vi "SPD.Config Read Test07 TR bifurcation.vi"(8 "Error In":errorcluster, 11 "SPD.Stand Ctrl in":T2 {"spdDeviceSession"."hidSPD.Sturtup Values"."HV_bias" format="%#_6p, V"; "spdDeviceSession"."hidSPD.Sturtup Values"."TSet" format="%#_6p, DegC"; "spdDeviceSession"."hidSPD.Controller"."HV_bias" format="%#_6p, V"; "spdDeviceSession"."hidSPD.Controller"."TSet" format="%#_6p, DegC"}) -> (0 "Error Out":errorcluster, 2 "TR_Bif Meas Params":T1, 3 "SPD.Stand Ctrl out":T2 {"spdDeviceSession"."hidSPD.Sturtup Values"."HV_bias" format="%#_6p, V"; "spdDeviceSession"."hidSPD.Sturtup Values"."TSet" format="%#_6p, DegC"; "spdDeviceSession"."hidSPD.Controller"."HV_bias" format="%#_6p, V"; "spdDeviceSession"."hidSPD.Controller"."TSet" format="%#_6p, DegC"})   [LabVIEW 2018]
uses:
  typedefs/SPD.Stand Ctrl.ctl
  Instruments/SPD HID Interface/hidSPDLibForLabView/LibVIs/hidSPD Controls/hidSPD Device Session.ctl
  Instruments/SPD HID Interface/hidSPDLibForLabView/LibVIs/hidSPD Controls/hidSPD Controller.ctl
  Instruments/SPD HID Interface/hidSPDLibForLabView/LibVIs/hidSPD Controls/hidSPD SPD Type.ctl
  Instruments/KC705 DevBoard/typedefs/DevB.Session.ctl
  Instruments/KeySight 53230A/typedefs/FreqC.Session.ctl
  Instruments/KeySight 8164B/KeySight 8164B LAN InstrLib/typedefs/KeySight 8164B control.ctl
  Instruments/LeCroy SDA830/typedefs/LeCroy.Session.ctl
  typedefs/SPD.Events.ctl
  SPD.Config File ctrl.ctl
  <vilib>/Utility/config.llb/Config Data RefNum.ctl
  typedefs/SPD.Meas Result.ctl
  typedefs/SPD.Queues.ctl
  typedefs/SPD.Stand state.ctl
  SPD Measurements/TR Bifurcation/typedefs/SPD.TR Test Params.ctl
  <vilib>/Utility/config.llb/Read Key (I32).vi
  <vilib>/Utility/config.llb/Read Key (Double).vi
  <vilib>/Utility/config.llb/Read Key (String).vi
  <vilib>/Utility/config.llb/NI_LVConfig.lvlib
  Instruments/KeySight 8164B/KeySight 8164B LAN InstrLib.lvlib
  Instruments/SPD HID Interface/hidSPDLibForLabView/hidSPDLibForLabView.lvlib
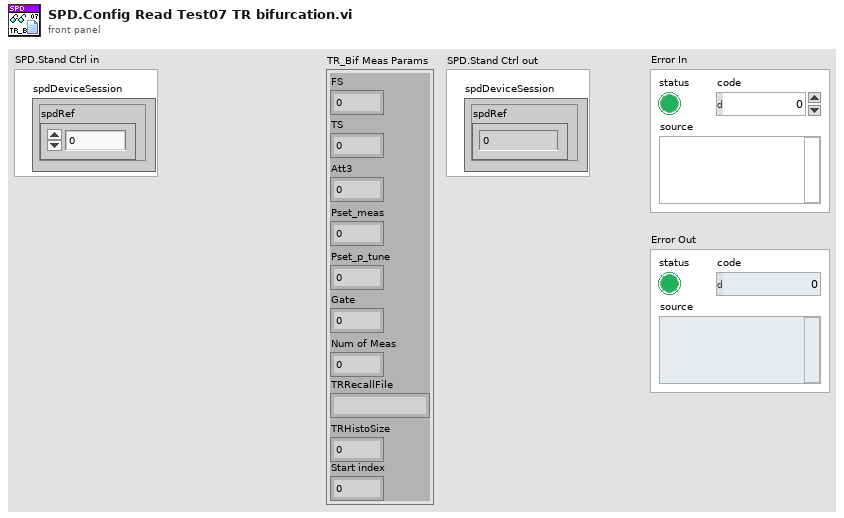
[diagram p1: front panel]
types:
  T1 = typedef "SPD.TR Test Params.ctl" = cluster{"FS":i32, "TS":i32, "Att3":dbl, "Pset_meas":dbl, "Pset_p_tune":dbl, "Gate":dbl, "Num of Meas":i32, "TRRecallFile":string, "TRHistoSize":i32, "Start index":i32}
  T2 = typedef "SPD.Stand Ctrl.ctl" = cluster{"spdDeviceSession":T3, "DevBSession":T6, "FreqCSession":T7, "8164BSession":T8, "LeCroySession":T9, "Events":T10, "configFile":T11, "SPD.Result":T13, "SPD.Queues":T14, "Console":refnum<vi>}
  T3 = typedef "hidSPDLibForLabView.lvlib/hidSPD Device Session.ctl" = cluster{"spdRef":u64, "connected":bool, "spdName":string, "hidSPD.Controller":T4, "hidSPD.Sturtup Values":T4, "SPD Type":T5}
  T4 = typedef "hidSPDLibForLabView.lvlib/hidSPD Controller.ctl" = cluster{"TSet":sgl, "HV_bias":sgl, "DDS_stb_code":u16}
  T5 = typedef "hidSPDLibForLabView.lvlib/hidSPD SPD Type.ctl" = enum16{"Free Run", "Gate"}
  T6 = typedef "DevB.Session.ctl" = cluster{"DevBRef":refnum<visa-resource-name>, "connected":bool}
  T7 = typedef "FreqC.Session.ctl" = cluster{"FreqCRef":refnum<visa-resource-name>, "timeout":dbl, "Gate":dbl, "connected":bool}
  T8 = typedef "KeySight 8164B LAN InstrLib.lvlib/KeySight 8164B control.ctl" = cluster{"Connection ID":refnum<k5>, "Connected":bool, "Info":string, "Slots Info":string[]}
  T9 = typedef "LeCroy.Session.ctl" = cluster{"LeCroySession":refnum<visa-resource-name>, "connected":bool}
  T10 = typedef "SPD.Events.ctl" = cluster{"DCRTest":refnum<user-event>, "Stop":refnum<user-event>}
  T11 = typedef "SPD.Config File ctrl.ctl" = cluster{"configFile ref":T12, "configFile path":path, "equipmentFile ref":T12}
  T12 = typedef "NI_LVConfig.lvlib/Config Data RefNum.ctl" = refnum<k1>
  T13 = typedef "SPD.Meas Result.ctl" = cluster{"HV_Bias":dbl[][][], "Stb_code":dbl[], "Temprature":dbl[], "Data":dbl[][][][], "DateTime":string}
  T14 = typedef "SPD.Queues.ctl" = cluster{"state queue":refnum<queue>}
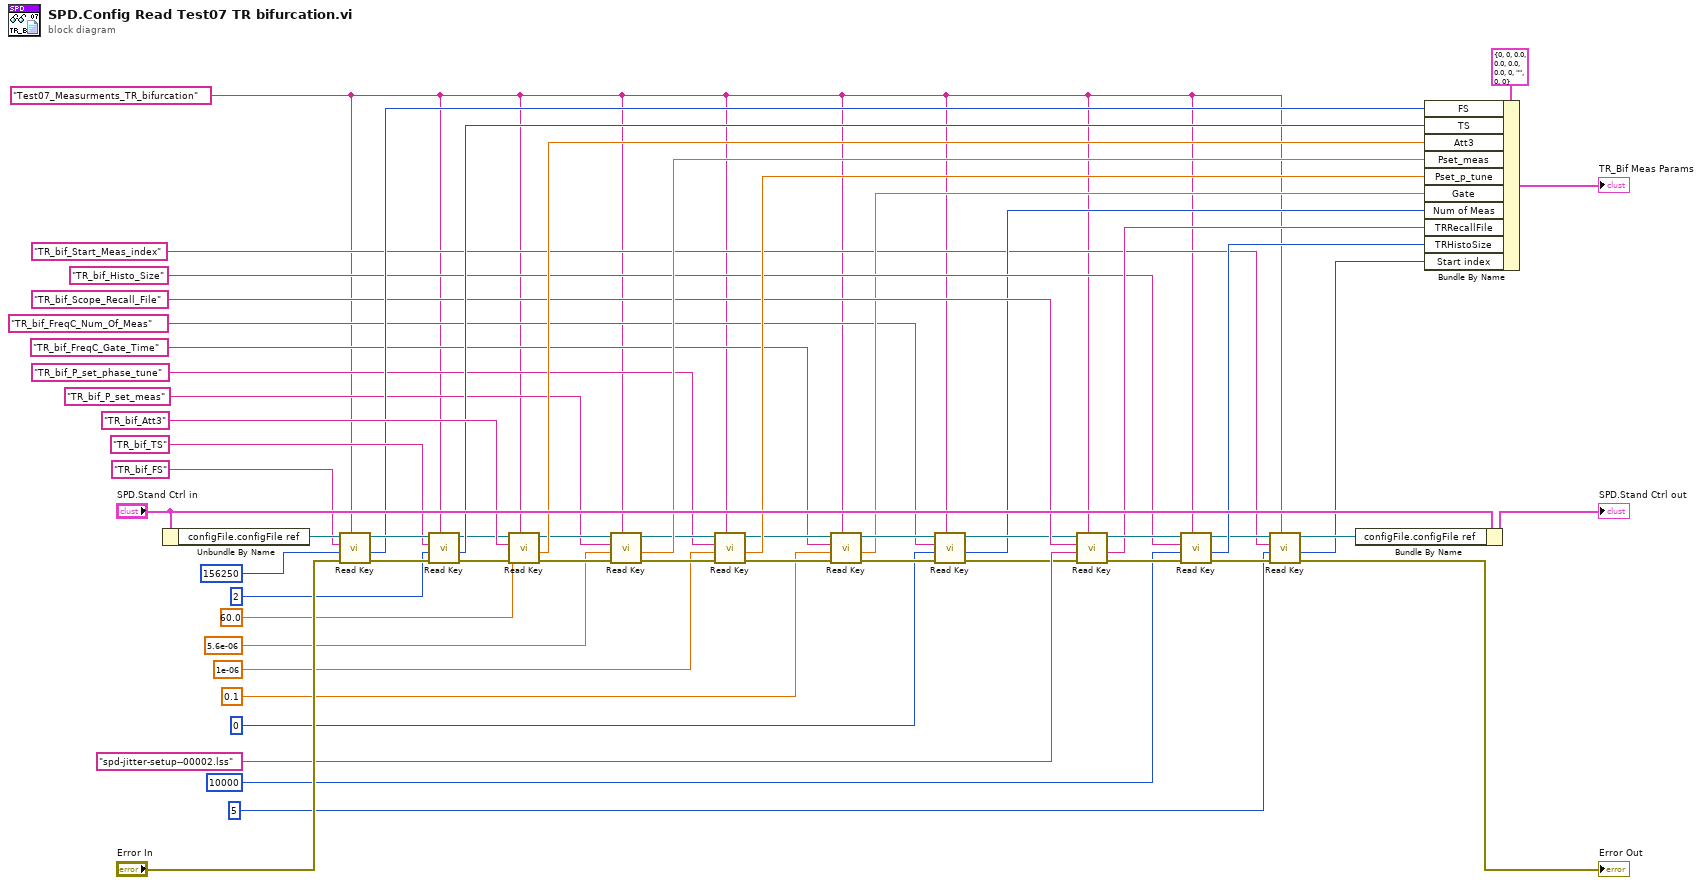
[diagram p0: block diagram]
diagram:
  w1 = "Test07_Measurments_TR_bifurcation" ("section")
  n1 = Unbundle By Name("SPD.Stand Ctrl in") -> ("configFile.configFile ref"=w55:T12)
  n2 = call-poly <vilib>:"Read Key.vi"("section"=w1, "error in (no error)"="Error In", "default value"=156250, "key"="TR_bif_FS", "refnum"=w55) -> ("error out"=w51:errorcluster, "value"=w45:i32, "refnum out"=w50:T12)  [unwired: 3 in, 1 out]
  n3 = call-poly <vilib>:"Read Key.vi"("section"=w1, "error in (no error)"=w51, "default value"=2, "key"="TR_bif_TS", "refnum"=w50) -> ("error out"=w35:errorcluster, "value"=w44:i32, "refnum out"=w36:T12)  [unwired: 3 in, 1 out]
  n4 = call-poly <vilib>:"Read Key.vi"("section"=w1, "error in (no error)"=w35, "default value"=60.0, "key"="TR_bif_Att3", "refnum"=w36) -> ("error out"=w40:errorcluster, "value"=w43:dbl, "refnum out"=w41:T12)  [unwired: 3 in, 1 out]
  n5 = call-poly <vilib>:"Read Key.vi"("section"=w1, "error in (no error)"=w40, "default value"=5.6e-06, "key"="TR_bif_P_set_meas", "refnum"=w41) -> ("error out"=w32:errorcluster, "value"=w39:dbl, "refnum out"=w33:T12)  [unwired: 3 in, 1 out]
  n6 = call-poly <vilib>:"Read Key.vi"("section"=w1, "error in (no error)"=w32, "default value"=1e-06, "key"="TR_bif_P_set_phase_tune", "refnum"=w33) -> ("error out"=w17:errorcluster, "value"=w29:dbl, "refnum out"=w18:T12)  [unwired: 3 in, 1 out]
  n7 = call-poly <vilib>:"Read Key.vi"("section"=w1, "error in (no error)"=w17, "default value"=0.1, "key"="TR_bif_FreqC_Gate_Time", "refnum"=w18) -> ("error out"=w20:errorcluster, "value"=w12:dbl, "refnum out"=w19:T12)  [unwired: 3 in, 1 out]
  n8 = call-poly <vilib>:"Read Key.vi"("section"=w1, "error in (no error)"=w20, "default value"=0, "key"="TR_bif_FreqC_Num_Of_Meas", "refnum"=w19) -> ("error out"=w16:errorcluster, "value"=w11:i32, "refnum out"=w15:T12)  [unwired: 3 in, 1 out]
  n9 = call-poly <vilib>:"Read Key.vi"("section"=w1, "error in (no error)"=w16, "default value"="spd-jitter-setup--00002.lss", "key"="TR_bif_Scope_Recall_File", "refnum"=w15) -> ("error out"=w27:errorcluster, "value"=w25:string, "refnum out"=w28:T12)  [unwired: 3 in, 1 out]
  n10 = call-poly <vilib>:"Read Key.vi"("section"=w1, "error in (no error)"=w27, "default value"=10000, "key"="TR_bif_Histo_Size", "refnum"=w28) -> ("error out"=w6:errorcluster, "value"=w23:i32, "refnum out"=w8:T12)  [unwired: 3 in, 1 out]
  n11 = call-poly <vilib>:"Read Key.vi"("section"=w1, "error in (no error)"=w6, "default value"=5, "key"="TR_bif_Start_Meas_index", "refnum"=w8) -> ("error out"=→"Error Out":errorcluster, "value"=w3:i32, "refnum out"=w7:T12)  [unwired: 3 in, 1 out]
  n12 = Bundle By Name(cluster="SPD.Stand Ctrl in", "configFile.configFile ref"=w7) -> (→"SPD.Stand Ctrl out":T2)
  n13 = Bundle By Name(cluster=T1 {"FS"=0, "TS"=0, "Att3"=0.0, "Pset_meas"=0.0, "Pset_p_tune"=0.0, "Gate"=0.0, "Num of Meas"=0, "TRRecallFile"="", "TRHistoSize"=0, "Start index"=0} ("APParams"), "FS"=w45, "TS"=w44, "Att3"=w43, "Pset_meas"=w39, "Pset_p_tune"=w29, "Gate"=w12, "Num of Meas"=w11, "TRRecallFile"=w25, "TRHistoSize"=w23, "Start index"=w3) -> (→"TR_Bif Meas Params":T1)
